vi "ADC_LTC1859_bitbang.vi"() -> ()   [LabVIEW 2015]
uses:
  <vilib>/myRIO/Instrument Drivers/Onboard IO/DIO/typedefs/DIO Reference.ctl
  <vilib>/myRIO/Common/Instrument Driver Framework/Utilities/typedefs/myRIO Generic Hardware Reference.ctl
  <vilib>/myRIO/Common/Instrument Driver Framework/Utilities/typedefs/Hardware Version Enum.ctl
  <vilib>/myRIO/Common/Instrument Driver Framework/Utilities/typedefs/myRIO v1.0 Reference.ctl
  <vilib>/myRIO/Common/Instrument Driver Framework/Utilities/typedefs/Generic FPGA Reference.ctl
  <vilib>/myRIO/Common/Instrument Driver Framework/myRIO v1.0/DIO/typedefs/DIO Channels List.ctl
  <vilib>/myRIO/Common/Instrument Driver Framework/myRIO v1.0/DIO/typedefs/DIO Channels Enum.ctl
  <vilib>/userdefined/High Color/nirio_resource_hc.ctl
  <vilib>/myRIO/Common/Instrument Driver Framework/Utilities/vis/Is FPGA Ref Available.vi
  <vilib>/myRIO/Common/Instrument Driver Framework/myRIO v1.0/DIO/vis/myRIO v1.1 Open DIO.vi
  <vilib>/myRIO/Instrument Drivers/Onboard IO/DIO/vis/Write.vi
  <vilib>/myRIO/Instrument Drivers/Onboard IO/DIO/vis/Read.vi
  <vilib>/myRIO/Common/Instrument Driver Framework/Utilities/vis/Validate Channels.vi
  <vilib>/myRIO/Common/Instrument Driver Framework/myRIO v1.0/DIO/vis/myRIO v1.0 Reserve DIO.vi
  <vilib>/myRIO/Common/Instrument Driver Framework/myRIO v1.0/Resource Manager/vis/myRIO v1.0 Reserve Channel List.vi
  <vilib>/myRIO/Common/Instrument Driver Framework/myRIO v1.0/DIO/vis/myRIO v1.0 Build MUX Configuration DIO.vi
  <vilib>/myRIO/Common/Instrument Driver Framework/myRIO v1.0/Resource Manager/vis/myRIO v1.0 Reserve Channel.vi
  <vilib>/myRIO/Common/Instrument Driver Framework/myRIO v1.0/Resource Manager/vis/myRIO v1.0 Unreserve Channel.vi
  <vilib>/myRIO/Common/Instrument Driver Framework/myRIO v1.0/Resource Manager/vis/myRIO v1.0 Create Configuration List.vi
  <vilib>/myRIO/Common/Instrument Driver Framework/myRIO v1.0/Resource Manager/vis/myRIO v1.0 Build Mutex Name.vi
  <vilib>/Utility/VariantDataType/GetNumericInfo.vi
  <vilib>/Utility/error.llb/Error Cluster From Error Code.vi
  <vilib>/myRIO/Common/Instrument Driver Framework/myRIO v1.0/myRIO v1.1 Open.vi
  <vilib>/myRIO/Common/Instrument Driver Framework/Utilities/vis/IO Manager.vi
  <vilib>/myRIO/Common/Instrument Driver Framework/Utilities/vis/Configuration Manager.vi
  <vilib>/myRIO/Common/Instrument Driver Framework/myRIO v1.0/Resource Manager/vis/myRIO v1.0 Configure IO.vi
  <vilib>/myRIO/Common/Instrument Driver Framework/myRIO v1.0/myRIO v1.0 Close.vi
  <vilib>/myRIO/Common/Instrument Driver Framework/myRIO v1.0/DIO/vis/myRIO v1.0 Write DIO.vi
  <vilib>/myRIO/Common/Instrument Driver Framework/myRIO v1.0/DIO/vis/myRIO v1.0 Read DIO.vi
  <vilib>/myRIO/Express VI/Onboard IO/DO/DO Express VI.xnode
  <vilib>/myRIO/Instrument Drivers/Onboard IO/DIO/vis/myRIO DIO Open.xnode
  <vilib>/myRIO/Express VI/Onboard IO/DI/DI Express VI.xnode
  <vilib>/myRIO/Instrument Drivers/Onboard IO/DIO/DIO.lvlib
panel:
  out "Array":bool[](array[boolean])
  out "Waveform Chart":dbl(graph)
  in  "Channel":dbl
  out "Sent":dbl[](array[numeric])
  in  "Pair":dbl
  in  "?":bool
  in  "?":bool
  # "Differential"
  # "single mode"
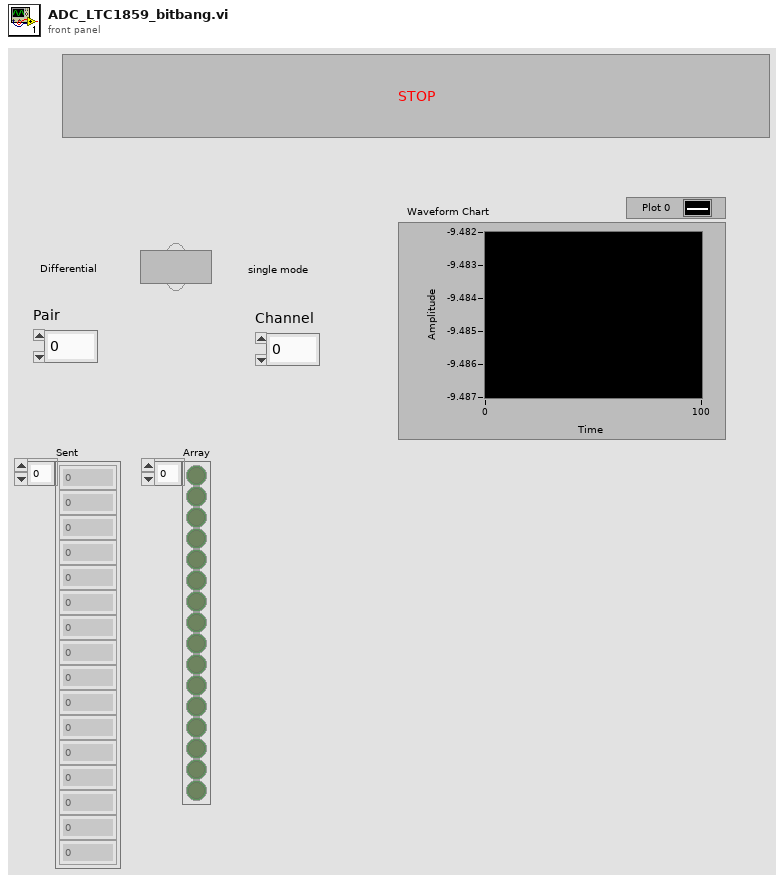
[diagram p1: front panel]
types:
  T1 = typedef "DIO.lvlib/DIO Reference.ctl" = cluster{"myRIO Reference":T2, "DIO Channels List":T6}
  T2 = typedef "myRIO Generic Hardware Reference.ctl" = cluster{"myRIO Model":T3, "myRIO Hardware Reference":T4}
  T3 = typedef "Hardware Version Enum.ctl" = enum16{"Unknown", "myRIO-1900", "myRIO-1950", "roboRIO"}
  T4 = typedef "myRIO v1.0 Reference.ctl" = cluster{"Generic FPGA Reference":T5, "Allow multiple opens":bool}
  T5 = typedef "Generic FPGA Reference.ctl" = refnum<k20>
  T6 = typedef "DIO Channels List.ctl" = T7[]
  T7 = typedef "DIO Channels Enum.ctl" = enum16{"Not Connected", "C/DIO0", "C/DIO1", "C/DIO2", "C/DIO3", "C/DIO4", "C/DIO5", "C/DIO6", "C/DIO7", "A/DIO0", "A/DIO1", "A/DIO2", "A/DIO3", "A/DIO4", "A/DIO5", "A/DIO6", "A/DIO7", "A/DIO8", "A/DIO9", "A/DIO10", "A/DIO11", "A/DIO12", "A/DIO13", "A/DIO14", "A/DIO15", "B/DIO0", "B/DIO1", "B/DIO2", "B/DIO3", "B/DIO4", "B/DIO5", "B/DIO6", "B/DIO7", "B/DIO8", "B/DIO9", "B/DIO10", "B/DIO11", "B/DIO12", "B/DIO13", "B/DIO14", "B/DIO15", "LED0", "LED1", "LED2", "LED3", "Button0", "DIO/DIO0", "DIO/DIO1", "DIO/DIO2", "DIO/DIO3", "DIO/DIO4", "DIO/DIO5", "DIO/DIO6", "DIO/DIO7", "DIO/DIO8", "DIO/DIO9", "SPI/CS0", "SPI/CS1", "SPI/CS2", "SPI/CS3", "LED RADIO (Green)", "LED RADIO (Red)", "LED COMM (Green)", "LED COMM (Red)", "LED MODE (Green)", "LED MODE (Red)"}
  T8 = typedef "nirio_resource_hc.ctl" = tag
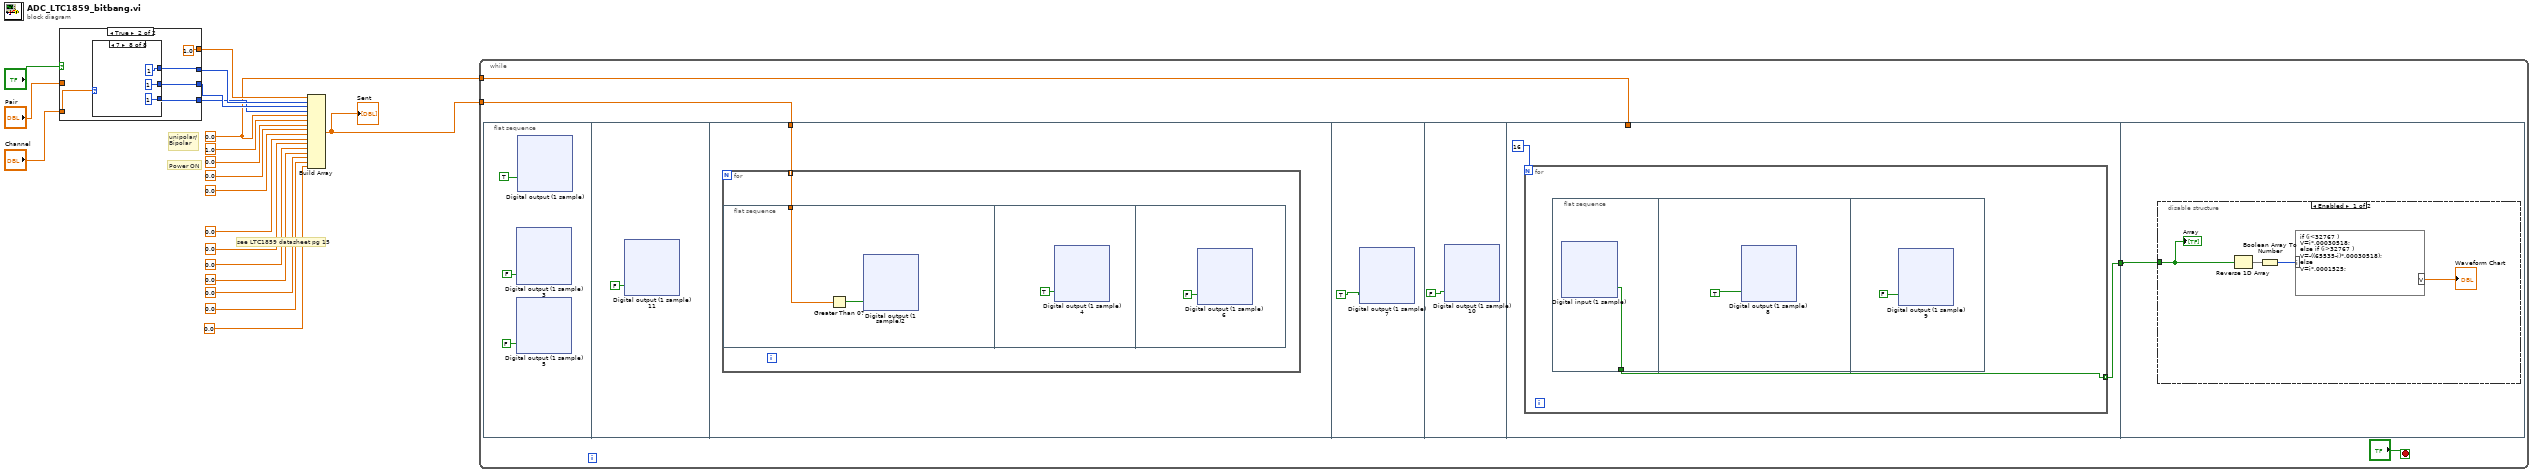
[diagram p0: block diagram]
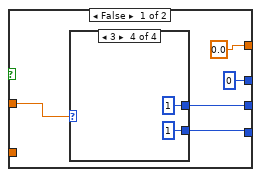
[diagram p2: hidden frame]
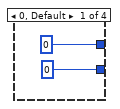
[diagram p3: hidden frame]
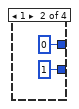
[diagram p4: hidden frame]
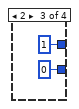
[diagram p5: hidden frame]
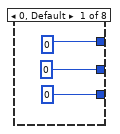
[diagram p6: hidden frame]
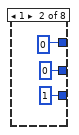
[diagram p7: hidden frame]
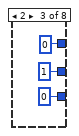
[diagram p8: hidden frame]
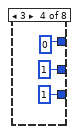
[diagram p9: hidden frame]
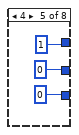
[diagram p10: hidden frame]
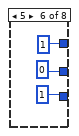
[diagram p11: hidden frame]
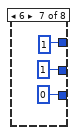
[diagram p12: hidden frame]
diagram:
  w2 = 0.0 ("element")
  # "see LTC1859 datasheet pg 15"
  # "Power ON"
  # "unipolar/\nBipolar"
  n1 = case shown="True" "?" {
    tunnel: [0.0 ("element") 1.0 ("element")] -> w3
    tunnel: "Pair" -> [w24 _]
    tunnel: "Channel" -> [_ w37]
    tunnel: [0 w36] -> w13
    tunnel: [w22 w35] -> w12
    tunnel: [w21 w34] -> w11
    frame False {
      n2 = case shown="3" w24 {
        tunnel: [0 0 1 1] -> w22
        tunnel: [0 1 0 1] -> w21
        frame 0, Default {
        }
        frame 1 {
        }
        frame 2 {
        }
        frame 3 {
        }
      }
    }
    frame True {
      n3 = case shown="7" w37 {
        tunnel: [0 0 1 1 0 0 1 1] -> w35
        tunnel: [0 1 0 1 0 1 0 1] -> w34
        tunnel: [0 0 0 0 1 1 1 1] -> w36
        frame 0, Default {
        }
        frame 1 {
        }
        frame 2 {
        }
        frame 3 {
        }
        frame 4 {
        }
        frame 5 {
        }
        frame 6 {
        }
        frame 7 {
        }
      }
    }
  }
  n4 = Build Array(w3, w13, w12, w11, w2, 1.0 ("element"), 0.0 ("element"), 0.0 ("element"), 0.0 ("element"), 0.0 ("element"), 0.0 ("element"), 0.0 ("element"), 0.0 ("element"), 0.0 ("element"), 0.0 ("element"), 0.0 ("element")) -> (w1:dbl[])
  "Sent" <- w1
  n5 = while {
    tunnel: w2 -> [w65]
    tunnel: w1 -> [w64]
    stop <- "?" stop-if-true
    n6 = flat-sequence {
      tunnel: w64 -> [w211]
      tunnel: w65 -> [_]
      tunnel: [w394] -> w63
      tunnel: w63 -> [w505]
      frame #0 {
        n7 = xnode "Digital output (1 sample) 5"("MOSI (A/DIO7 (Pin 25))"=FALSE) -> ()  [unwired: 1 in, 1 out]
        n8 = xnode "Digital output (1 sample) 3"("Clock (A/DIO5 (Pin 21))"=FALSE) -> ()  [unwired: 1 in, 1 out]
        n9 = xnode "Digital output (1 sample)"("CS (A/DIO0 (Pin 11))"=TRUE ("A/DIO0 (Pin 11)")) -> ()  [unwired: 1 in, 1 out]
      }
      frame #1 {
        n10 = xnode "Digital output (1 sample) 11"("CS (A/DIO0 (Pin 11))"=FALSE) -> ()  [unwired: 1 in, 1 out]
      }
      frame #2 {
        n11 = for {
          tunnel: w211 -> [w212] mode=indexing
          n12 = flat-sequence {
            tunnel: w212 -> [w213]
            frame #0 {
              n13 = Greater Than 0?(x=w213) -> (x > 0?=w214:bool)
              n14 = xnode "Digital output (1 sample)2"("MOSI (A/DIO7 (Pin 25))"=w214) -> ()  [unwired: 1 in, 1 out]
            }
            frame #1 {
              n15 = xnode "Digital output (1 sample) 4"("Clock (A/DIO5 (Pin 21))"=TRUE) -> ()  [unwired: 1 in, 1 out]
            }
            frame #2 {
              n16 = xnode "Digital output (1 sample) 6"("Clock (A/DIO5 (Pin 21))"=FALSE) -> ()  [unwired: 1 in, 1 out]
            }
          }
        }
      }
      frame #3 {
        n17 = xnode "Digital output (1 sample) 7"("CS (A/DIO0 (Pin 11))"=TRUE ("A/DIO0 (Pin 11)")) -> ()  [unwired: 1 in, 1 out]
      }
      frame #4 {
        n18 = xnode "Digital output (1 sample) 10"("CS (A/DIO0 (Pin 11))"=FALSE ("A/DIO0 (Pin 11)")) -> ()  [unwired: 1 in, 1 out]
      }
      frame #5 {
        n19 = for {
          N: 16 -> [_]
          tunnel: [w396] -> w394 mode=indexing
          n20 = flat-sequence {
            tunnel: [w397] -> w396
            frame #0 {
              n21 = xnode "Digital input (1 sample)"() -> ("MISO (A/DIO6 (Pin 23))"=w397:bool)  [unwired: 1 in, 1 out]
            }
            frame #1 {
              n22 = xnode "Digital output (1 sample) 8"("Clock (A/DIO5 (Pin 21))"=TRUE) -> ()  [unwired: 1 in, 1 out]
            }
            frame #2 {
              n23 = xnode "Digital output (1 sample) 9"("Clock (A/DIO5 (Pin 21))"=FALSE) -> ()  [unwired: 1 in, 1 out]
            }
          }
        }
      }
      frame #6 {
        n24 = disable-structure shown="Enabled" {
          disable-tunnel: w505 -> [w507 _]
          frame Enabled {
            n25 = Reverse 1D Array(array=w507) -> (reversed array=w506:bool[])
            n26 = Boolean Array To Number(Boolean array=w506) -> (number=w508:u32)
            n27 = formula code="if (i<32767 )\nV=i*.00030518;\nelse if (i>32767 )\nV=-((65535-i)*.00030518);\nelse\nV=i*.0001525;"("i"=w508) -> ("V"=→"Waveform Chart":dbl)
            "Array" <- w507
          }
          frame Disabled {
          }
        }
      }
    }
  }
